vi "appendParagraph.vi"(8 "error in (no error)":errorcluster, 10 "paragraph":refnum<k24>, 11 "XWPFDocuement in":refnum<k24>) -> (0 "error out":errorcluster, 3 "XWPFDocuement out":refnum<k24>)   [LabVIEW 2017, in "LabVIEW NPOI.lvlib" / "xwpfWriter.lvclass"]
uses:
  xwpfWriter.lvclass
  C:/Users/Neo/Desktop/Dev_Tools_BR/LabVIEW_NPOI/lib/NPOI 2.1.1/NPOI.OOXML.dll
  lib/NPOI 2.1.1/NPOI.OOXML.dll
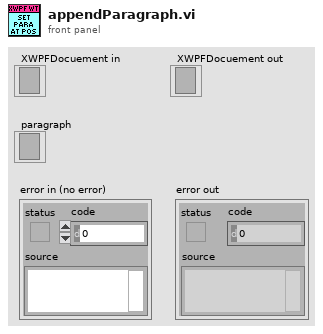
[diagram p1: front panel]
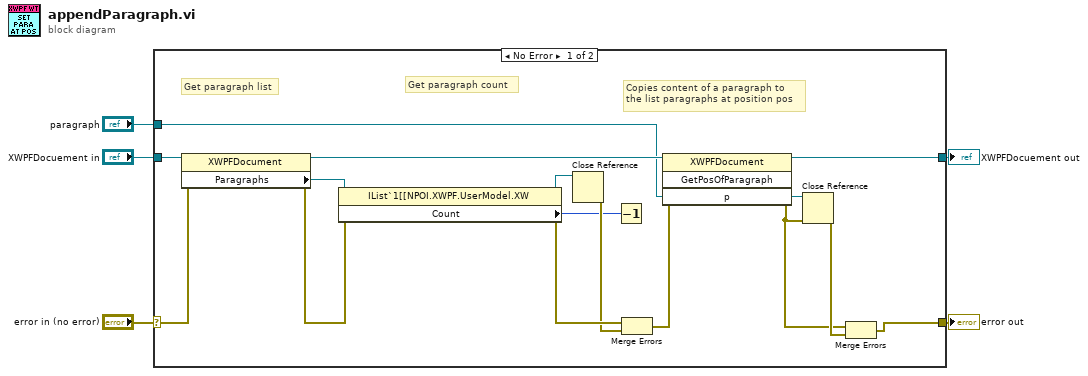
[diagram p0: block diagram]
diagram:
  n1 = case shown="No Error" "error in (no error)" {
    selector: "error in (no error)" -> [w19 w21]
    tunnel: [w10 w21] -> w4
    tunnel: "XWPFDocuement in" -> [w14 _]
    tunnel: [w12 _] -> w2
    tunnel: "paragraph" -> [w6 _]
    frame No Error {
      # "Copies content of a paragraph to \nthe list paragraphs at position pos"
      # "Get paragraph count"
      # "Get paragraph list"
      n2 = property class="XWPFDocument"(reference=w14, error in=w19) -> (reference out=w13:refnum<k24>, error out=w18:errorcluster, "Paragraphs"=w20:refnum<k24>)
      n3 = property class="IList`1[[NPOI.XWPF.UserModel.XW"(reference=w20, error in=w18) -> (reference out=w17:refnum<k24>, error out=w16:errorcluster, "Count"=w7:i32)
      n4 = Close Reference(reference=w17) -> (error out=w15:errorcluster)  [unwired: 1 in]
      n5 = Decrement(x=w7) -> ()  [unwired: 1 out]
      n6 = Merge Errors(w16, w15) -> (w11:errorcluster)
      n7 = invoke class="XWPFDocument" method="GetPosOfParagraph"(reference=w13, error in=w11, "p"=w6) -> (reference out=w12:refnum<k24>, error out=w8:errorcluster)  [unwired: 1 in, 2 out]
      n8 = Close Reference(reference=w6, error in (no error)=w8) -> (error out=w9:errorcluster)
      n9 = Merge Errors(w8, w9) -> (w10:errorcluster)
    }
    frame Error {
    }
  }
  "error out" <- w4
  "XWPFDocuement out" <- w2
